vi "OpenVS(Silent).vi"   [LabVIEW 2011]
uses:
  <vilib>/Utility/sysdir.llb/System Directory Type.ctl
panel:
  # "This VI calls VS silently"
types:
  T1 = typedef "System Directory Type.ctl" = i32
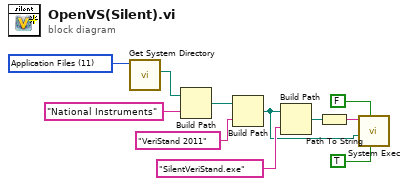
[diagram p0: block diagram]
diagram:
  w9 = T1 11 items=["User Home"=0, "User Desktop"=1, "User Documents"=2, "User Application Data"=3, "User Preferences"=4, "User Temporary"=5, "Public Documents"=6, "Public Application Data"=7, "Public Preferences"=8, "Public Cache"=13, "System Core Libraries"=9, "System Installed Libraries"=10, "Application Files"=11, "Boot Volume Root"=12] ("system directory type")
  n1 = call <vilib>:"Get System Directory.vi"("system directory type"=w9) -> ("system directory"=w8:path)  [unwired: 10 in]
  n2 = Build Path(base path=w8, name or relative path="National Instruments") -> (appended path=w6:path)
  n3 = Build Path(base path=w6, name or relative path="VeriStand 2011") -> (appended path=w1:path)
  n4 = Build Path(base path=w1, name or relative path="SilentVeriStand.exe") -> (appended path=w3:path)
  n5 = Path To String(path=w3) -> (string=w2:string)
  n6 = call <vilib>:"System Exec.vi"("run minimized? (F)"=TRUE, "wait until completion? (T)"=FALSE, "working directory"=w1, "command line"=w2) -> ()  [unwired: 4 in, 4 out]
